vi "Filter Packets.vi"(10 "Boolean":bool, 11 "LiveData in":T1 {"Reference/Temperature 2" format="%.2f"; "Accelerometer" format="%.2f"; "Battery" format="%.2f"; "Reference/Temperature" format="%.2f"; "LoadSensors" format="%.2f"}) -> (3 "LiveData out":T1 {"Reference/Temperature 2" format="%.2f"; "Accelerometer" format="%.2f"; "Battery" format="%.2f"; "Reference/Temperature" format="%.2f"; "LoadSensors" format="%.2f"})   [LabVIEW 2013]
uses:
  Controls/LiveData.ctl
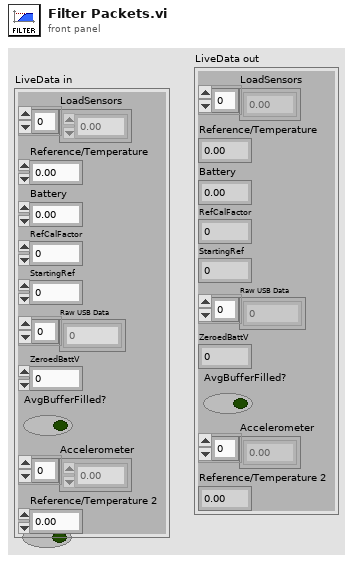
[diagram p1: front panel]
types:
  T1 = typedef "LiveData.ctl" = cluster{"LoadSensors":dbl[], "Reference/Temperature":dbl, "Battery":dbl, "RefCalFactor":dbl, "StartingRef":dbl, "Raw USB Data":u16[], "ZeroedBattV":dbl, "AvgBufferFilled?":bool, "Accelerometer":dbl[], "Reference/Temperature 2":dbl}
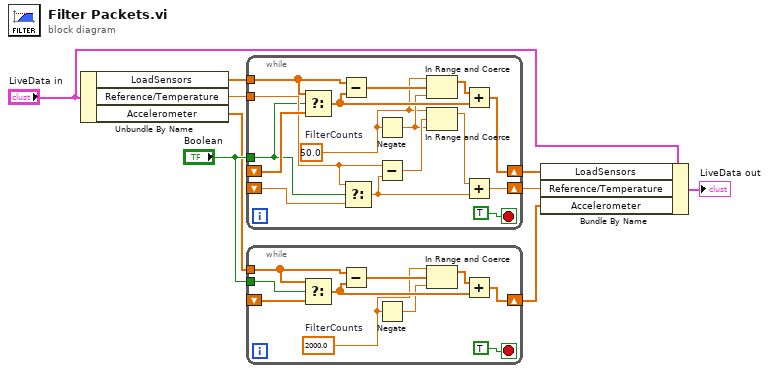
[diagram p0: block diagram]
diagram:
  n1 = Unbundle By Name("LiveData in") -> ("LoadSensors"=w2:dbl[], "Reference/Temperature"=w3:dbl, "Accelerometer"=w7:dbl[])
  n2 = while {
    shift-right: [w20] -> w5
    shift-left: _ -> [w22]
    tunnel: w2 -> [w21]
    shift-right: [w19] -> w6
    shift-left: _ -> [w17]
    tunnel: w3 -> [w18]
    tunnel: "Boolean" -> [w12]
    stop <- TRUE stop-if-true
    w10 = 50.0  # FilterCounts
    n3 = Select(t=w21, s=w12, f=w22) -> (s? t:f=w23:dbl[])
    n4 = Subtract(x=w21, y=w23) -> (x-y=w25:dbl[])
    n5 = Select(t=w18, s=w12, f=w17) -> (s? t:f=w16:dbl)
    n6 = Negate(x=w10) -> (-x=w11:dbl)
    n7 = Subtract(x=w18, y=w16) -> (x-y=w14:dbl)
    n8 = In Range and Coerce(upper limit=w10, x=w25, lower limit=w11) -> (coerced(x)=w24:dbl[])  [unwired: 1 out]
    n9 = In Range and Coerce(upper limit=w10, x=w14, lower limit=w11) -> (coerced(x)=w15:dbl)  [unwired: 1 out]
    n10 = Add(x=w24, y=w23) -> (x+y=w20:dbl[])
    n11 = Add(x=w15, y=w16) -> (x+y=w19:dbl)
  }
  n12 = while {
    shift-right: [w31] -> w9
    shift-left: _ -> [w32]
    tunnel: "Boolean" -> [w29]
    tunnel: w7 -> [w26]
    stop <- TRUE stop-if-true
    w27 = 2000.0  # FilterCounts
    n13 = Select(t=w26, s=w29, f=w32) -> (s? t:f=w33:dbl[])
    n14 = Subtract(x=w26, y=w33) -> (x-y=w35:dbl[])
    n15 = Negate(x=w27) -> (-x=w28:dbl)
    n16 = In Range and Coerce(upper limit=w27, x=w35, lower limit=w28) -> (coerced(x)=w34:dbl[])  [unwired: 1 out]
    n17 = Add(x=w34, y=w33) -> (x+y=w31:dbl[])
  }
  n18 = Bundle By Name(cluster="LiveData in", "LoadSensors"=w5, "Reference/Temperature"=w6, "Accelerometer"=w9) -> (→"LiveData out":T1)
